vi "Scroll_Pump_Test.vi"() -> ()   [LabVIEW 2014]
uses:
  <vilib>/NI/STM/TCP/TCP Data Info.ctl
  C:/Program Files (x86)/National Instruments/LabVIEW 2014/examples/Data Communication/Network Streams/Simple Network Streams/support/Network Stream Command.ctl
  <vilib>/dex/Stream Element Allocation Mode.ctl
  <vilib>/Platform/TimedLoop/XDataNode/timing_clust.ctl
  <vilib>/Platform/TimedLoop/XDataNode/nitl_modes.ctl
  <vilib>/Platform/TimedLoop/XDataNode/wakeup.ctl
  <vilib>/NI/STM/TCP/Read Meta Data (TCP Ref).vi
  <vilib>/NI/STM/TCP/Get Connection Reference (TCP).vi
  <vilib>/NI/STM/TCP/Read Meta Data (TCP Clst).vi
  <vilib>/NI/STM/TCP/Read Message (TCP).vi
  <vilib>/platform/TimedLoop/XDataNode/XDataNode.xnode
  <vilib>/Platform/TimedLoop/XDataNode/XDNodeRunTimeDep.lvlib
  <vilib>/NI/STM/NI STM.lvlib
panel:
  in  "Standby Speed %\nDefault Set Value":u32=66 min=66 max=100
  out "error out 2":errorcluster
  in  "Normal Speed threshold":u32(slide)=50 min=50 max=100 scale=50.0..100.0
  out "Message Count\ndata info":T1
  out "Array 4":errorcluster[](array[cluster])
  out "Array 3":string[](array[string])
  out "Array 2":bool[](array[boolean])
  in  "Target IP Address":string="192.168.101.17"
  out "Fault register":bool[](array[boolean])
  out "Warning register":bool[](array[boolean])
  out "System status register 2":bool[](array[boolean])
  out "System status register":bool[](array[boolean])
  out "Motor Frequency":i32(graph)
  out "Measured Motor Power (W)":dbl(knob) scale=0.0..800.0
  out "Measured Link Voltage (V)":dbl(knob) scale=0.0..800.0
  out "Measured Motor Current (A)":dbl(knob) scale=0.0..6.0
  out "Pump Temperature":i32(slide) scale=-500.0..100.0
  out "Pump Controller Temperature":i32(slide) scale=0.0..100.0
  out "Receiver Loop Count":i32
  in  "Standby Speed threshold\n66% - 100%":u32=66 min=66 max=100
  in  "Use Standby Speed":bool
  in  "Pump On/Off":bool
  out "FGGA command sender error out":errorcluster
  # "Stop command received and pump is stopping"
  # "Power limit is active"
  # "Accelerating / running"
  # "Acceleration is limited"
  # "Standby Active"
  # "Deceleration is limited"
  # "Above normal speed"
  # "Operating above the ramp speed threshold"
  # "Operating above the overload speed threshold"
  # "Control mode"
  # "Warning Condition"
  # "Fault Condition"
  # "Serial enable active"
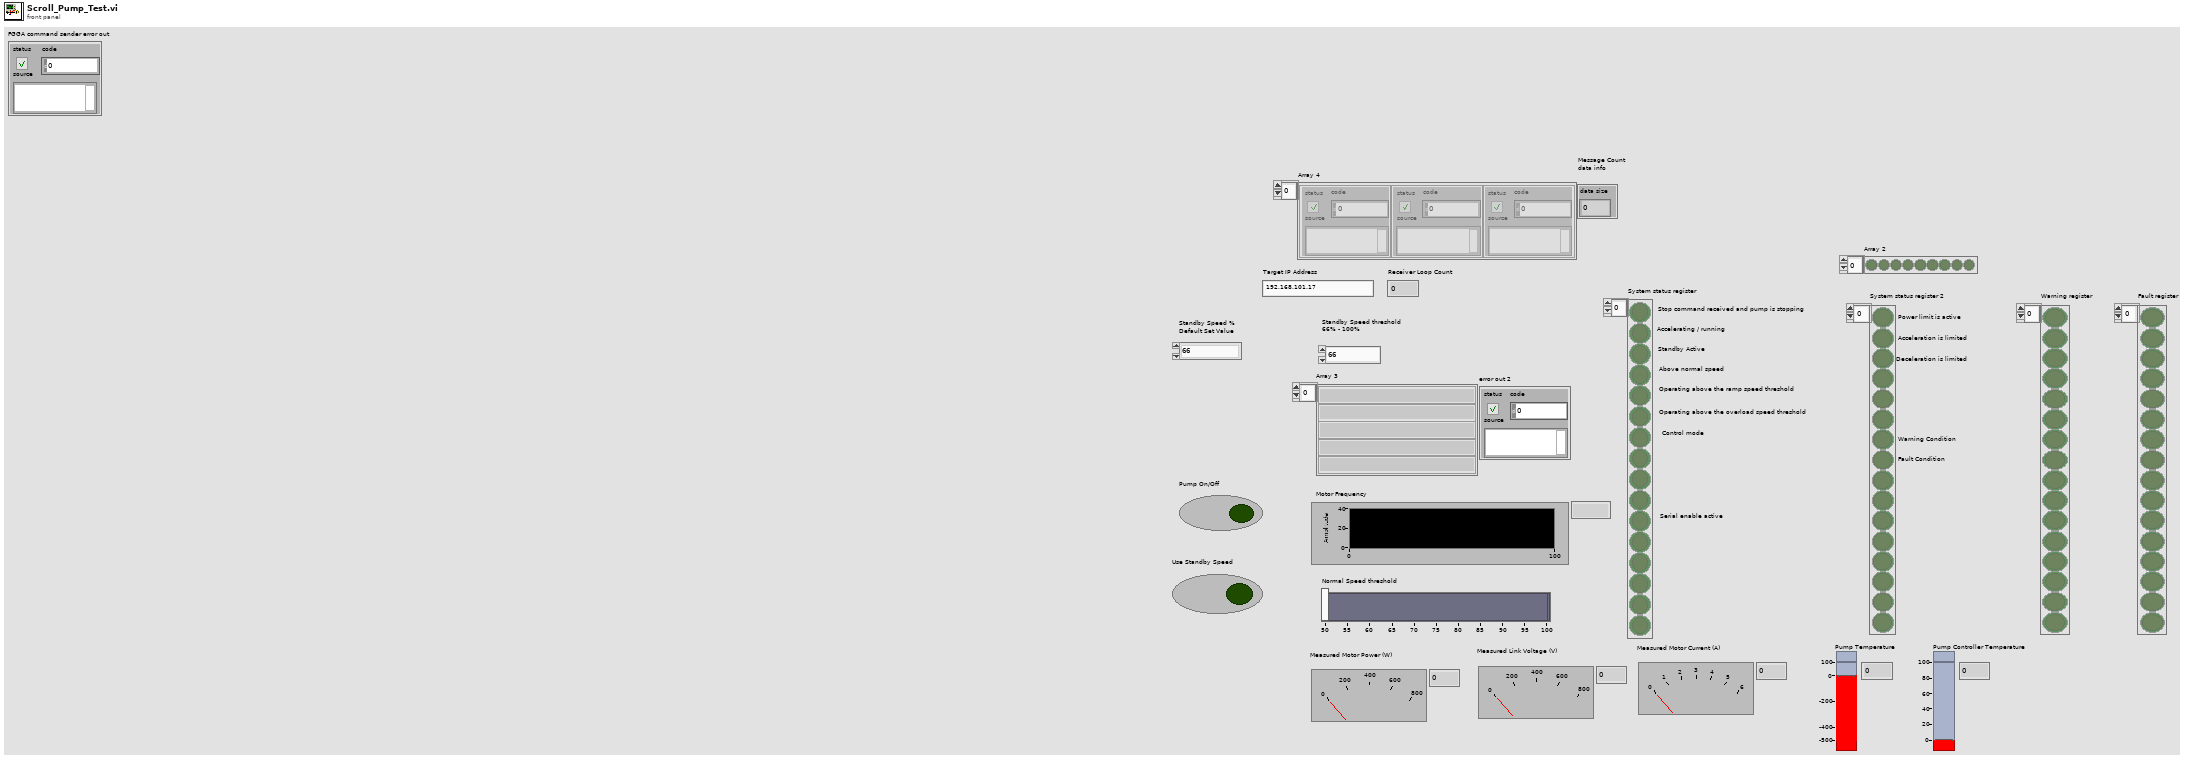
[diagram p1: front panel]
types:
  T1 = typedef "NI STM.lvlib/TCP Data Info.ctl" = cluster{"data size":i32}
  T2 = typedef "Stream Element Allocation Mode.ctl" = u32
  T3 = typedef "Network Stream Command.ctl" = cluster{"Message":string, "Message Data":variant}
  T4 = typedef "XDNodeRunTimeDep.lvlib/timing_clust.ctl" = cluster{"Expected End [f-1]":u64, "Actual End [f-1]":u64, "Finished Late? [f-1]":bool, "Expected End [i-1]":u64, "Actual End [i-1]":u64, "Finished Late? [i-1]":bool, "Expected Start [i]":u64, "Actual Start [i]":u64, "Expected Start [f]":u64, "Actual Start [f]":u64, "Source Name":string, "Structure Name":string, "Period":i64, "Deadline":i64, "Offset":i64, "Start":i64, "Priority":i32, "Timeout":i32, "Mode":T5, "Wakeup Reason":T6, "Error":errorcluster, "Source Type":string, "Secondary Source Type":string, "Global End Time":u64, "Global Start Time":u64, "Frame Duration":u64, "Iteration Duration":u64, "Assigned CPU":i32, "I/O Scan Engine Mode":u32}
  T5 = typedef "XDNodeRunTimeDep.lvlib/nitl_modes.ctl" = enum32{"No Change", "Process missed periods, maintain original phase", "Discard missed periods, maintain original phase", "Process missed periods, ignore original phase", "Discard missed periods, ignore original phase"}
  T6 = typedef "XDNodeRunTimeDep.lvlib/wakeup.ctl" = enum32{"Normal", "Aborted", "Asynchronous wakeup", "Timing source error", "Timed loop error", "Timeout"}
  T7 = typedef "NI STM.lvlib/TCP Connection Info.ctl" = cluster{"connection ID":refnum<k5>, "meta data":T8[]}
  T8 = typedef "NI STM.lvlib/MetaDataElement.ctl" = string
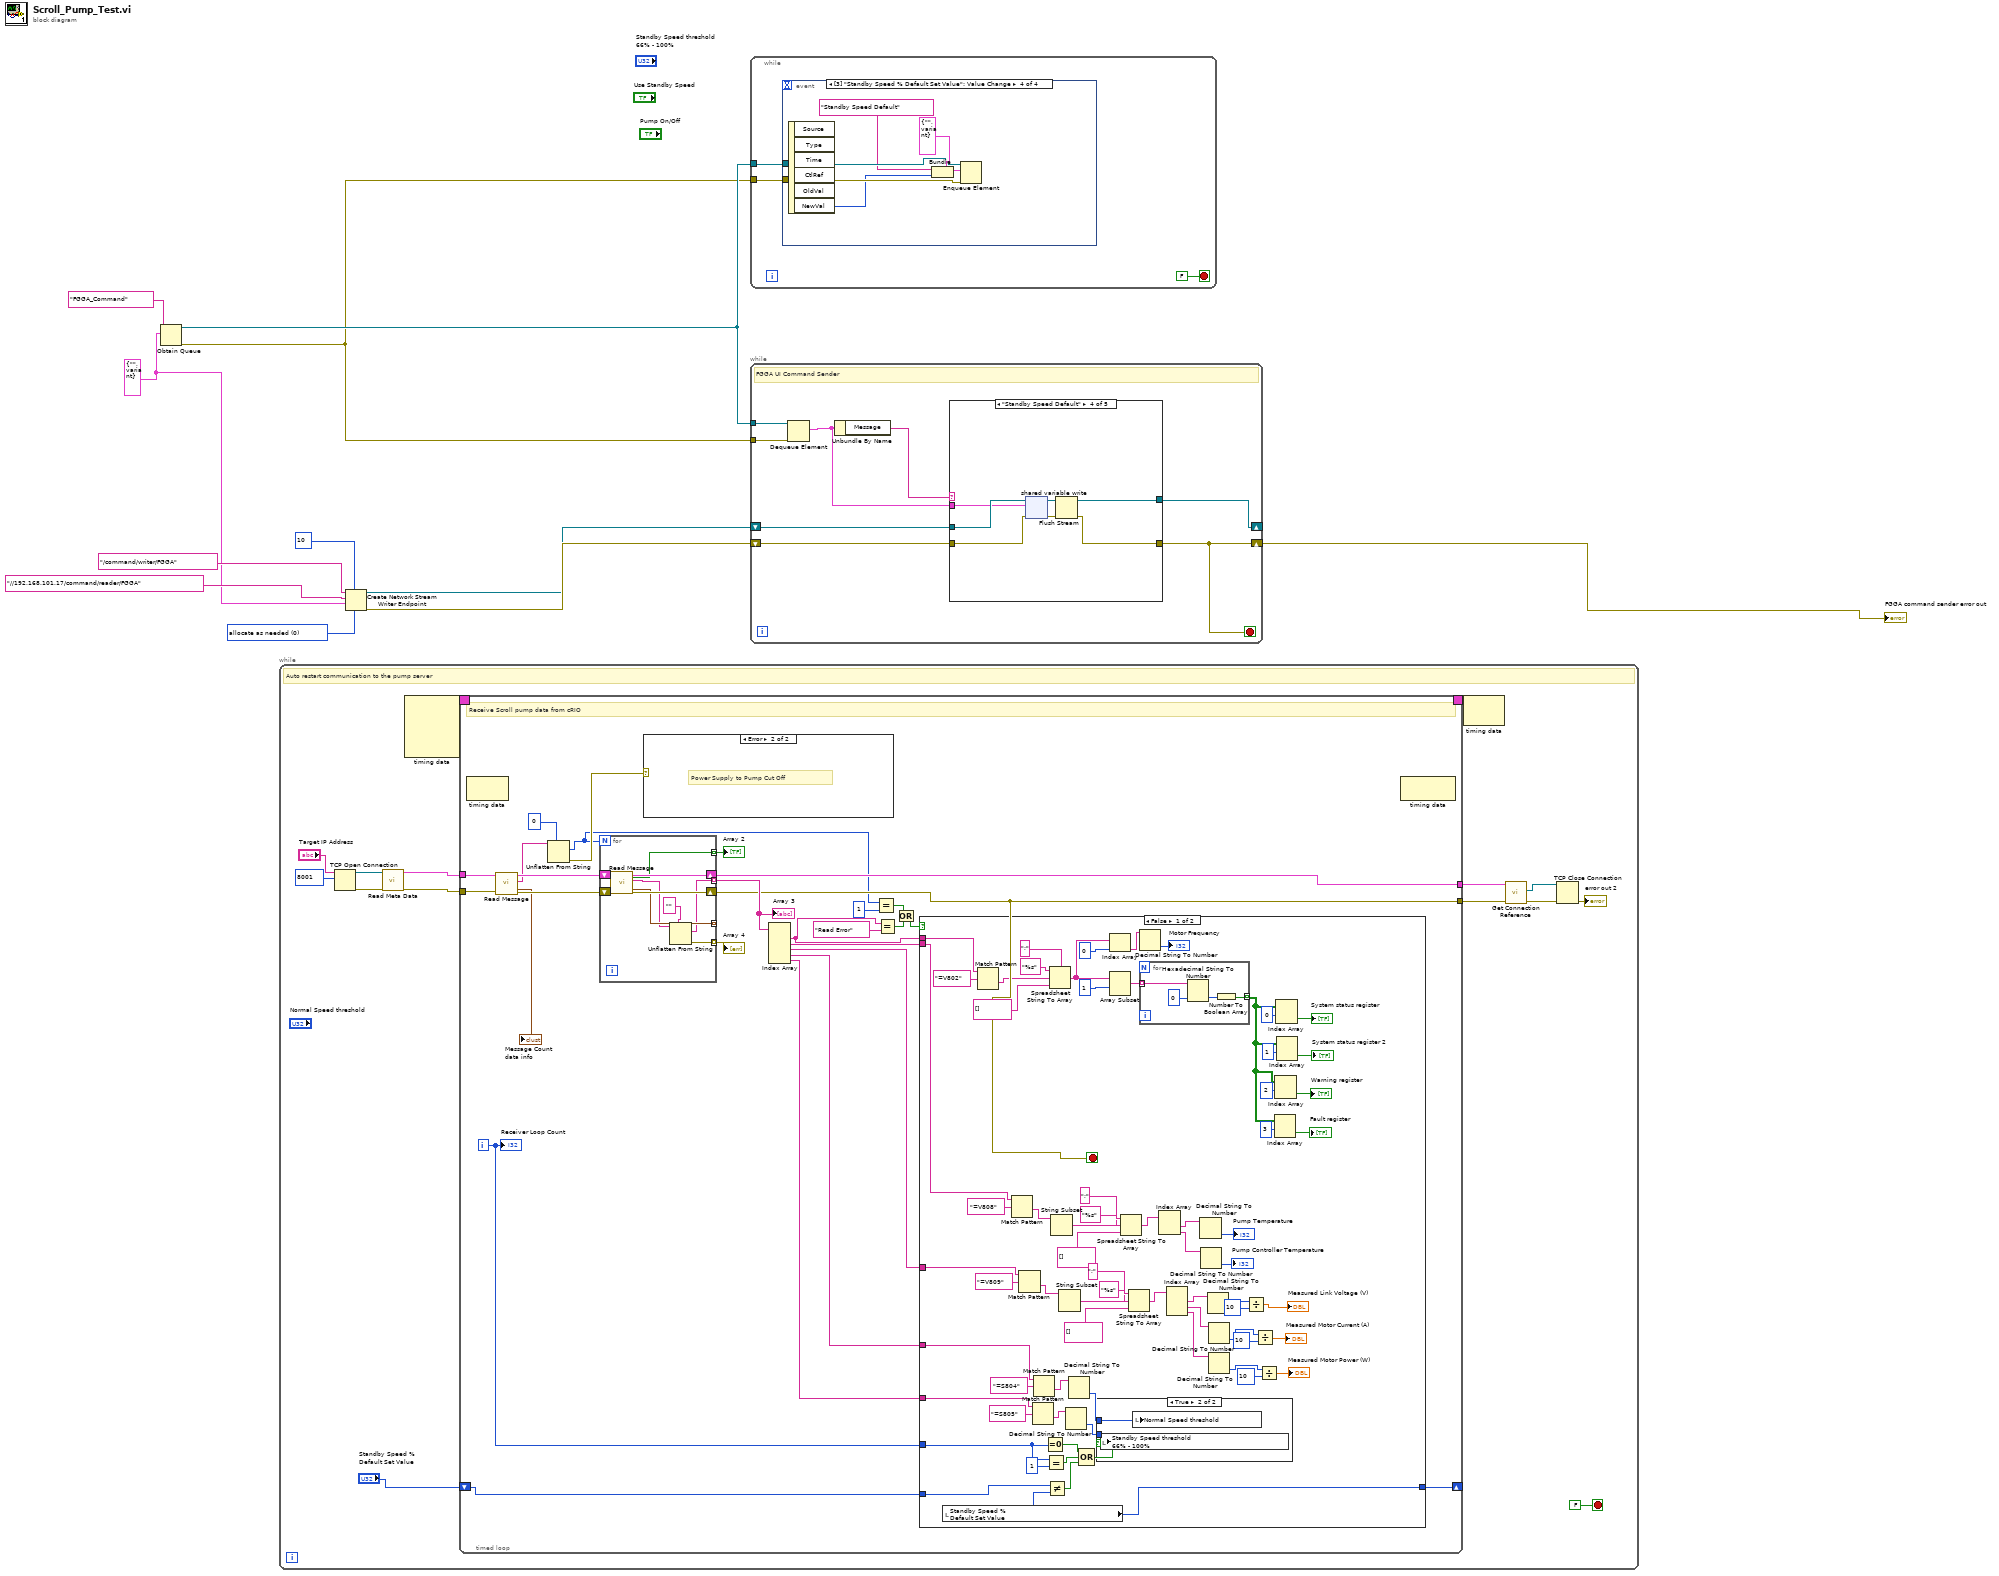
[diagram p0: block diagram]
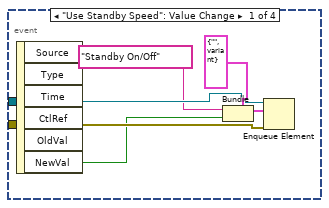
[diagram p5: hidden frame]
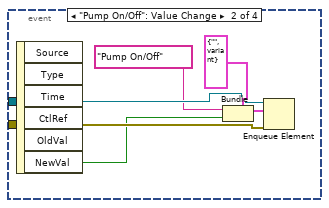
[diagram p6: hidden frame]
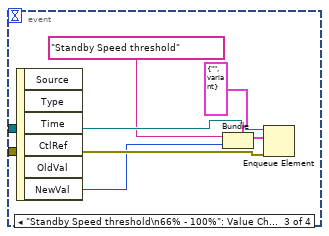
[diagram p7: hidden frame]
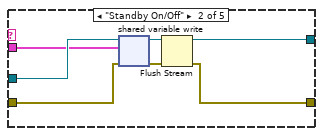
[diagram p9: hidden frame]
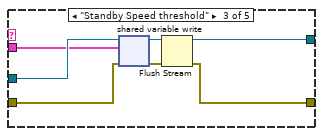
[diagram p10: hidden frame]
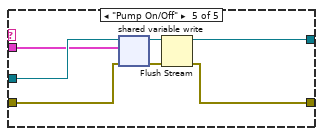
[diagram p11: hidden frame]
diagram:
  w8 = T2 0 items=["allocate as needed", "pre-allocate"] ("element allocation mode")
  w3 = T3 {"Message"="", "Message Data"=variant} ("Message Cluster")
  n1 = Obtain Queue(name (unnamed)="FGGA_Command", element data type=w3) -> (queue out=w2:refnum<queue>, error out=w1:errorcluster)  [unwired: 3 in, 1 out]
  n2 = while {
    stop <- FALSE stop-if-true
    # "Auto restart communication to the pump server"
    n3 = TCP Open Connection(address="Target IP Address", remote port or service name=u16 8001 ("remote port")) -> (connection ID=w24:refnum<k5>, error out=w23:errorcluster)  [unwired: 1 in, 2 out]
    n4 = call-poly <vilib>:"Read Meta Data.vi"("error in"=w23, "connection ID"=w24) -> ("error out"=w19:errorcluster, "connection info out"=w20:T7)  [unwired: 1 in, 7 out]
    n5 = node-c288() -> (w26:T4)  [unwired: 4 in]
    n6 = timed-loop {
      timing: w26 -> [_]
      timing-out: [_] -> w25
      tunnel: w20 -> [w44]
      tunnel: w19 -> [w47]
      tunnel: [w53] -> w17
      tunnel: [w38] -> w16
      shift-right: [w27] -> _
      shift-left: "Standby Speed %\nDefault Set Value" -> [w28]
      i -> [w37]
      stop <- w38 stop-if-true
      # "Receive Scroll pump data from cRIO"
      n7 = node-c288() -> ()  [unwired: 1 in, 1 out]
      n8 = call-poly <vilib>:"Read Message.vi"("error in"=w47, "connection info in"=w44) -> ("error out"=w46:errorcluster, "data string"=w42:string, "connection info out"=w45:T7, "data info"=→"Message Count\ndata info":T1)  [unwired: 1 in, 5 out]
      n9 = Unflatten From String(type=0, binary string=w42) -> (value=w32:i32, error out=w36:errorcluster)  [unwired: 1 in, 3 out]
      n10 = for {
        N: w32 -> [_]
        shift-right: [w137] -> w53
        shift-left: w45 -> [w139]
        shift-right: [w136] -> w38
        shift-left: w46 -> [w138]
        tunnel: [w135] -> _ mode=indexing
        tunnel: [w131] -> w52 mode=indexing
        tunnel: [w134] -> w51 mode=indexing
        tunnel: [w130] -> w48 mode=indexing
        n11 = call-poly <vilib>:"Read Message.vi"("error in"=w138, "connection info in"=w139) -> ("error out"=w136:errorcluster, "data string"=w132:string, "connection info out"=w137:T7, "data info"=w135:T1, "timed out?"=w134:bool)  [unwired: 1 in, 4 out]
        n12 = Unflatten From String(type="", binary string=w132) -> (value=w131:string, error out=w130:errorcluster)  [unwired: 1 in, 3 out]
      }
      "Array 2" <- w51
      "Array 3" <- w52
      "Array 4" <- w48
      n13 = case shown="Error" w36 {
        frame No Error {
        }
        frame Error {
          # "Power Supply to Pump Cut Off"
        }
      }
      n14 = Index Array(array=w52) -> (element #1=w35:string, element #2=w50:string, element #3=w49:string, element #4=w40:string, element #5=w39:string)  [unwired: 5 in]
      n15 = Equal?(x=w32, y=1) -> (x = y?=w31:bool)
      n16 = Equal?(x=w35, y="Read Error") -> (x = y?=w30:bool)
      n17 = Or(x=w31, y=w30) -> (x .or. y?=w29:bool)
      n18 = case shown="False" w29 {
        tunnel: w35 -> [w72 _]
        tunnel: w50 -> [w71 _]
        tunnel: w49 -> [w70 _]
        tunnel: w40 -> [w65 _]
        tunnel: w39 -> [w64 _]
        tunnel: w37 -> [w61 _]
        tunnel: w28 -> [w56 w129]
        tunnel: [w54 w129] -> w27
        frame False {
          n19 = local read "Standby Speed %\nDefault Set Value"() -> (w54:u32)
          n20 = Match Pattern(string=w72, regular expression="=V802") -> (after substring=w73:string)  [unwired: 1 in, 3 out]
          n21 = Match Pattern(string=w71, regular expression="=V808") -> (after substring=w117:string)  [unwired: 1 in, 3 out]
          n22 = Match Pattern(string=w70, regular expression="=V809") -> (after substring=w106:string)  [unwired: 1 in, 3 out]
          n23 = Match Pattern(string=w64, regular expression="=S805") -> (after substring=w66:string)  [unwired: 1 in, 3 out]
          n24 = Match Pattern(string=w65, regular expression="=S804") -> (after substring=w67:string)  [unwired: 1 in, 3 out]
          n25 = Equal To 0?(x=w61) -> (x = 0?=w59:bool)
          n26 = Equal?(x=w61, y=1) -> (x = y?=w60:bool)
          n27 = Not Equal?(x=w56, y=w54) -> (x != y?=w55:bool)
          n28 = Spreadsheet String To Array(delimiter (Tab)=";", format string="%s", spreadsheet string=w73, array type (2D Dbl)=string[] []) -> (array=w87:string[])
          n29 = String Subset(string=w117) -> (substring=w119:string)  [unwired: 2 in]
          n30 = String Subset(string=w106) -> (substring=w108:string)  [unwired: 2 in]
          n31 = Decimal String To Number(string=w66) -> (number=w63:i32)  [unwired: 2 in, 1 out]
          n32 = Decimal String To Number(string=w67) -> (number=w62:i32)  [unwired: 2 in, 1 out]
          n33 = Compound Arithmetic op=OR(w59, w60, w55) -> (w58:bool)
          n34 = case shown="True" w58 {
            tunnel: w63 -> [_ w124]
            tunnel: w62 -> [_ w123]
            frame False {
            }
            frame True {
              n35 = local write "Standby Speed threshold\n66% - 100%"(w124) -> ()
              n36 = local write "Normal Speed threshold"(w123) -> ()
            }
          }
          n37 = Index Array(array=w87, index=0) -> (element=w85:string)
          n38 = Array Subset(array=w87, index=1) -> (w88:string[])  [unwired: 1 in]
          n39 = Spreadsheet String To Array(delimiter (Tab)=";", format string="%s", spreadsheet string=w119, array type (2D Dbl)=string[] []) -> (array=w116:string[])
          n40 = Spreadsheet String To Array(delimiter (Tab)=";", format string="%s", spreadsheet string=w108, array type (2D Dbl)=string[] []) -> (array=w105:string[])
          n41 = Decimal String To Number(string=w85) -> (number=→"Motor Frequency":i32)  [unwired: 2 in, 1 out]
          n42 = for {
            tunnel: w88 -> [w128] mode=indexing
            tunnel: [w125] -> w75 mode=indexing
            n43 = Hexadecimal String To Number(string=w128, default (0uL)=u16 0 ("default (0 U32)")) -> (number=w126:u16)  [unwired: 1 in, 1 out]
            n44 = Number To Boolean Array(number=w126) -> (Boolean array=w125:bool[])
          }
          n45 = Index Array(array=w116) -> (element #1=w115:string, element #2=w113:string)  [unwired: 2 in]
          n46 = Index Array(array=w105) -> (element #1=w104:string, element #2=w103:string, element #3=w102:string)  [unwired: 3 in]
          n47 = Decimal String To Number(string=w115) -> (number=→"Pump Temperature":i32)  [unwired: 2 in, 1 out]
          n48 = Decimal String To Number(string=w113) -> (number=→"Pump Controller Temperature":i32)  [unwired: 2 in, 1 out]
          n49 = Decimal String To Number(string=w104) -> (number=w101:i32)  [unwired: 2 in, 1 out]
          n50 = Decimal String To Number(string=w103) -> (number=w97:i32)  [unwired: 2 in, 1 out]
          n51 = Decimal String To Number(string=w102) -> (number=w94:i32)  [unwired: 2 in, 1 out]
          n52 = Divide(x=w101, y=10) -> (x/y=→"Measured Link Voltage (V)":dbl)
          n53 = Divide(x=w97, y=10) -> (x/y=→"Measured Motor Current (A)":dbl)
          n54 = Divide(x=w94, y=10) -> (x/y=→"Measured Motor Power (W)":dbl)
          n55 = Index Array(array=w75, index (row)=3) -> (element=→"Fault register":bool[])  [unwired: 1 in]
          n56 = Index Array(array=w75, index (row)=2) -> (element=→"Warning register":bool[])  [unwired: 1 in]
          n57 = Index Array(array=w75, index (row)=0) -> (element=→"System status register":bool[])  [unwired: 1 in]
          n58 = Index Array(array=w75, index (row)=1) -> (element=→"System status register 2":bool[])  [unwired: 1 in]
        }
        frame True {
        }
      }
      n59 = node-c288() -> ()  [unwired: 1 in, 1 out]
      "Receiver Loop Count" <- w37
    }
    n60 = node-c288(w25) -> ()  [unwired: 1 out]
    n61 = call-poly <vilib>:"Get Connection Reference.vi"("error in"=w16, "connection info in"=w17) -> ("error out"=w18:errorcluster, "connection ID out"=w15:refnum<k5>)  [unwired: 8 out]
    n62 = TCP Close Connection(connection ID=w15, error in (no error)=w18) -> (error out=→"error out 2":errorcluster)  [unwired: 2 out]
  }
  n63 = Create Network Stream Writer Endpoint(6:w8, 7:10 ("writer buffer size"), 9:w3, 10:"//192.168.101.17/command/reader/FGGA" ("reader url"), 11:"/command/writer/FGGA" ("writer name")) -> (0:w7:errorcluster, 3:w6:refnum<k21>)  [unwired: 2 in]
  n64 = while {
    tunnel: w2 -> [w151]
    shift-right: [w146] -> _
    shift-left: w6 -> [w148]
    shift-right: [w144] -> w4
    shift-left: w7 -> [w150]
    tunnel: w1 -> [w145]
    stop <- w144 stop-if-true
    # "FGGA UI Command Sender"
    n65 = Dequeue Element(queue=w151, error in (no error)=w145) -> (element=w147:T3)  [unwired: 1 in, 3 out]
    n66 = Unbundle By Name(w147) -> ("Message"=w149:string)
    n67 = case shown="\"Standby Speed Default\"" w149 {
      tunnel: w150 -> [w152 w156 w163 w170 w177]
      tunnel: w148 -> [w153 w159 w166 w173 w180]
      tunnel: w147 -> [_ w158 w165 w172 w179]
      tunnel: [w152 w155 w162 w169 w176] -> w144
      tunnel: [w153 w154 w161 w168 w175] -> w146
      frame "False", Default {
      }
      frame "Standby On/Off" {
        n68 = shared-variable-write(w159, w156, w158) -> (w157:refnum<k21>, w160:errorcluster)  [unwired: 1 in, 1 out]
        n69 = Flush Stream(8:w160, 11:w157) -> (0:w155:errorcluster, 3:w154:refnum<k21>)  [unwired: 2 in, 1 out]
      }
      frame "Standby Speed threshold" {
        n70 = shared-variable-write(w166, w163, w165) -> (w164:refnum<k21>, w167:errorcluster)  [unwired: 1 in, 1 out]
        n71 = Flush Stream(8:w167, 11:w164) -> (0:w162:errorcluster, 3:w161:refnum<k21>)  [unwired: 2 in, 1 out]
      }
      frame "Standby Speed Default" {
        n72 = shared-variable-write(w173, w170, w172) -> (w171:refnum<k21>, w174:errorcluster)  [unwired: 1 in, 1 out]
        n73 = Flush Stream(8:w174, 11:w171) -> (0:w169:errorcluster, 3:w168:refnum<k21>)  [unwired: 2 in, 1 out]
      }
      frame "Pump On/Off" {
        n74 = shared-variable-write(w180, w177, w179) -> (w178:refnum<k21>, w181:errorcluster)  [unwired: 1 in, 1 out]
        n75 = Flush Stream(8:w181, 11:w178) -> (0:w176:errorcluster, 3:w175:refnum<k21>)  [unwired: 2 in, 1 out]
      }
    }
  }
  "FGGA command sender error out" <- w4
  n76 = while {
    tunnel: w2 -> [w184]
    tunnel: w1 -> [w183]
    stop <- FALSE stop-if-true
    n77 = event shown="[3] \"Standby Speed % Default Set Value\": Value Change" {
      selector: _ -> [_ _ _ _]
      dyn-events: _ -> [_ _ _ _]
      timeout: _ -> [_ _ _ _]
      tunnel: w184 -> [w188 w194 w200 w206]
      tunnel: w183 -> [w187 w193 w199 w205]
      event "Use Standby Speed": Value Change {
        n78 = event-data() -> ("NewVal"=w185:bool)  [unwired: 1 in, 5 out]
        n79 = Bundle(cluster=T3 {"Message"="", "Message Data"=variant} ("Message Cluster"), "Message"="Standby On/Off", "Message Data"=w185) -> (w189:T3)
        n80 = Enqueue Element(queue=w188, element=w189, error in (no error)=w187) -> ()  [unwired: 1 in, 3 out]
      }
      event "Pump On/Off": Value Change {
        n81 = event-data() -> ("NewVal"=w191:bool)  [unwired: 1 in, 5 out]
        n82 = Bundle(cluster=T3 {"Message"="", "Message Data"=variant} ("Message Cluster"), "Message"="Pump On/Off", "Message Data"=w191) -> (w195:T3)
        n83 = Enqueue Element(queue=w194, element=w195, error in (no error)=w193) -> ()  [unwired: 1 in, 3 out]
      }
      event "Standby Speed threshold\n66% - 100%": Value Change {
        n84 = event-data() -> ("NewVal"=w197:u32)  [unwired: 1 in, 5 out]
        n85 = Bundle(cluster=T3 {"Message"="", "Message Data"=variant} ("Message Cluster"), "Message"="Standby Speed threshold", "Message Data"=w197) -> (w201:T3)
        n86 = Enqueue Element(queue=w200, element=w201, error in (no error)=w199) -> ()  [unwired: 1 in, 3 out]
      }
      event "Standby Speed %\nDefault Set Value": Value Change {
        n87 = event-data() -> ("NewVal"=w203:u32)  [unwired: 1 in, 5 out]
        n88 = Bundle(cluster=T3 {"Message"="", "Message Data"=variant} ("Message Cluster"), "Message"="Standby Speed Default", "Message Data"=w203) -> (w207:T3)
        n89 = Enqueue Element(queue=w206, element=w207, error in (no error)=w205) -> ()  [unwired: 1 in, 3 out]
      }
    }
  }
